vi "Examen2 (2).vi"() -> ()   [LabVIEW 2018]
uses:
  EstadosExamen2.ctl
panel:
  out "Indicador Distancia Recorrida":i32
  out "Indicador Zona Aleatoria":i32
  out "Indicador Nectar Tomado 3":i32(slide) caption="Indicador Salud" scale=0.0..10.0
  out "Indicador Nectar Tomado 2":i32(slide) caption="Indicador Dosis\n       Disponibles" scale=0.0..20.0
  out "Mosca Zona 3":bool
  out "Mosca Zona 2":bool
  out "Mosca Zona 1":bool
  in  "Control Salta":bool
  in  "Control Zona":i32(slide) scale=1.0..3.0
  out "Indicador Zona":i32
  out "Indicador Nectar Tomado":i32(slide) caption="Indicador Nectar\n       Tomado" scale=0.0..5.0
  in  "Control Nectar":bool
  in  "stop":bool
  out "Indicador Estado":T1
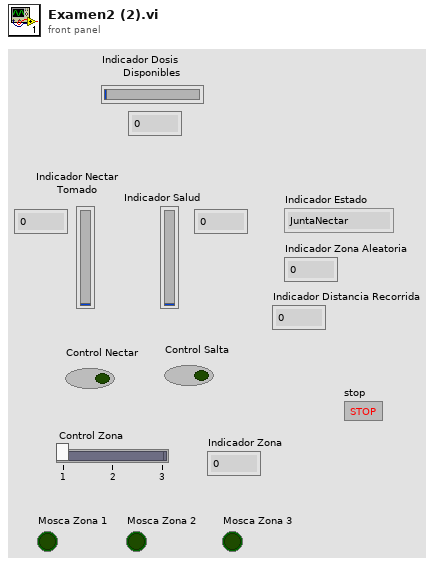
[diagram p1: front panel]
types:
  T1 = typedef "EstadosExamen2.ctl" = enum16{"JuntaNectar", "Volando", "Zona 1", "Zona 2", "Zona 3"}
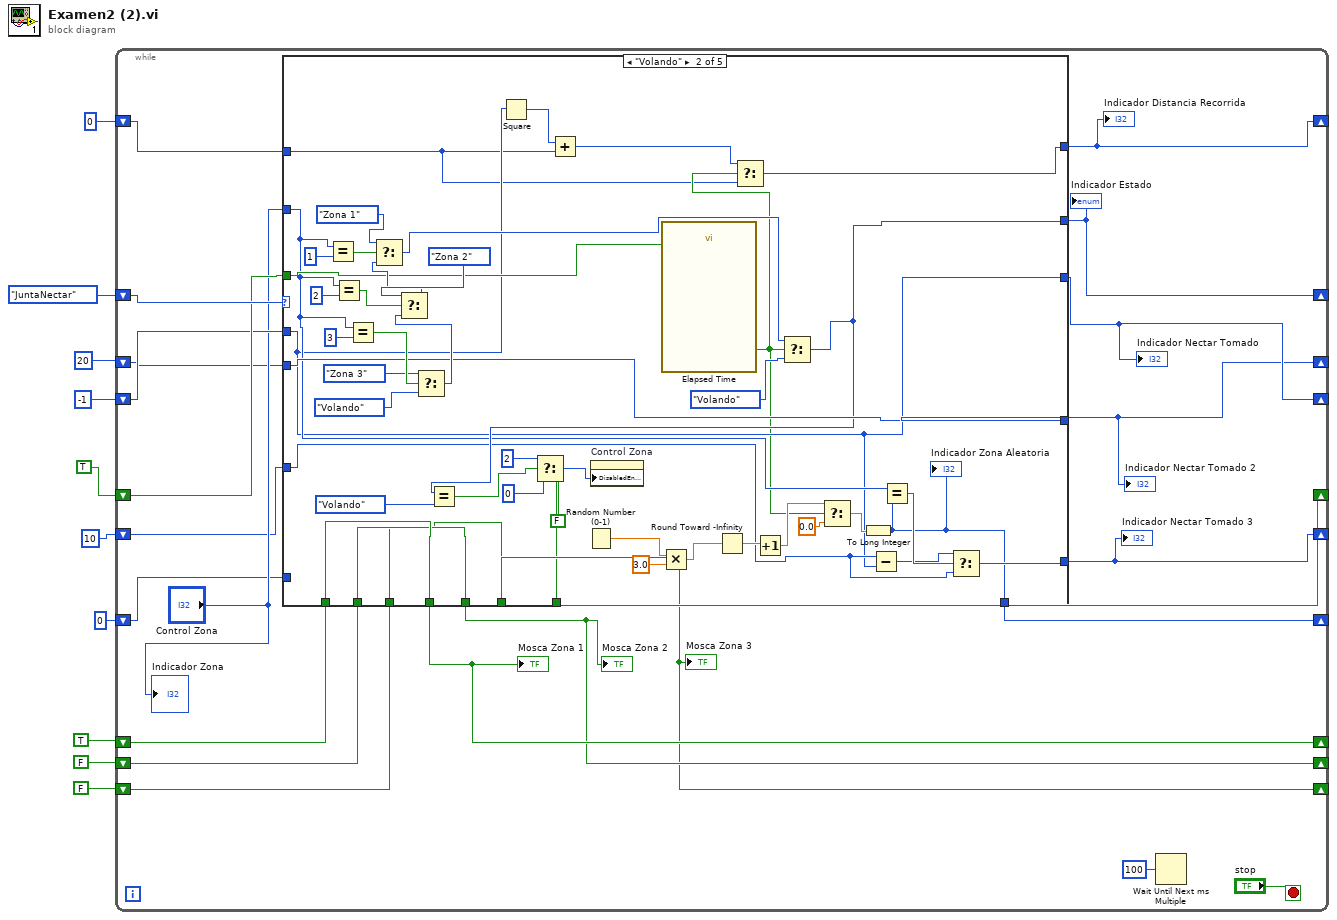
[diagram p0: block diagram]
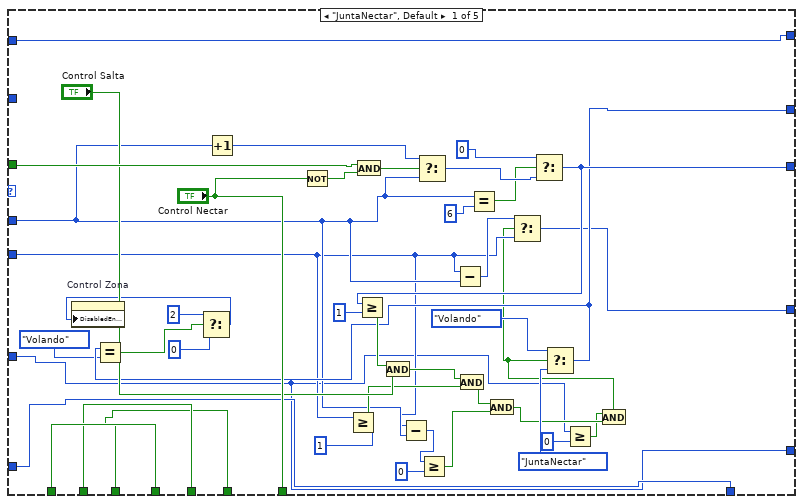
[diagram p2: hidden frame]
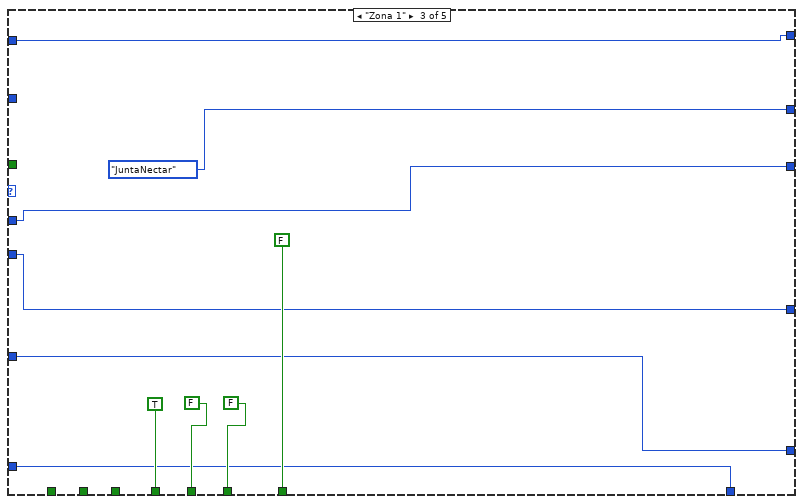
[diagram p3: hidden frame]
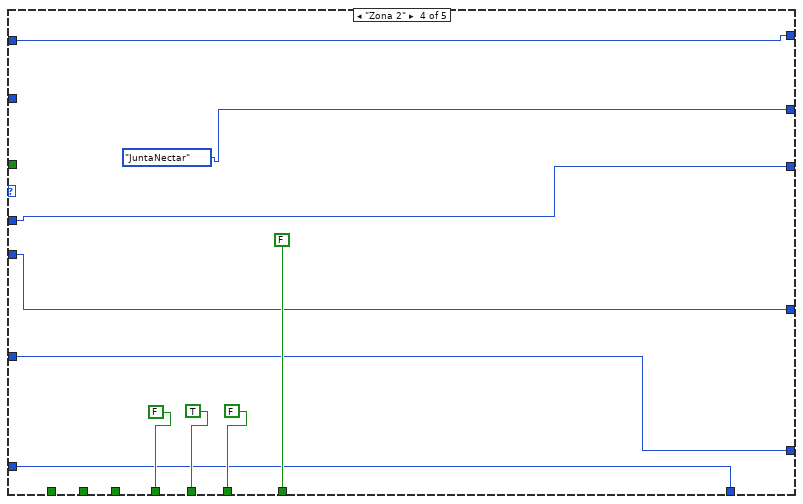
[diagram p4: hidden frame]
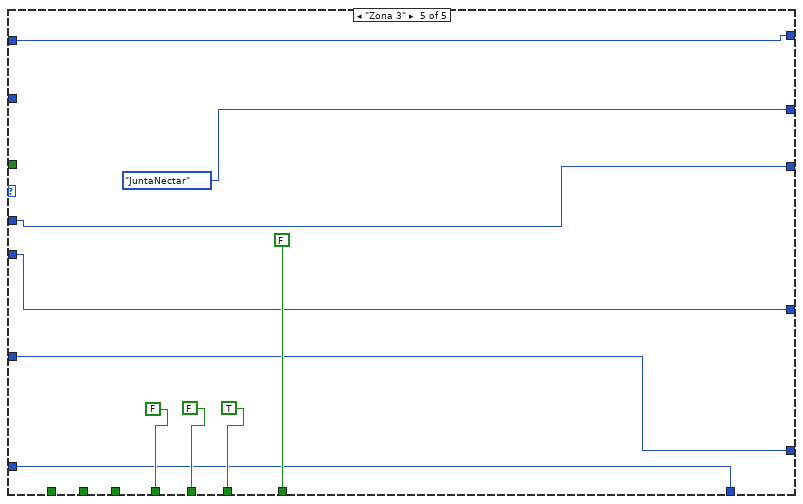
[diagram p5: hidden frame]
diagram:
  n1 = while {
    shift-right: [w32] -> _
    shift-left: EstadosExamen2."JuntaNectar" -> [w33]
    shift-right: [w27] -> _
    shift-left: -1 -> [w26]
    shift-right: [w29] -> _
    shift-left: TRUE -> [w28]
    shift-right: [w21] -> _
    shift-left: TRUE -> [w24]
    shift-right: [w20] -> _
    shift-left: FALSE -> [w23]
    shift-right: [w19] -> _
    shift-left: FALSE -> [w22]
    shift-right: [w18] -> _
    shift-left: 20 -> [w17]
    shift-right: [w15] -> _
    shift-left: 10 -> [w16]
    shift-right: [w14] -> _
    shift-left: 0 -> [w13]
    shift-right: [w11] -> _
    shift-left: 0 -> [w12]
    stop <- "stop" stop-if-true
    n2 = case shown="\"Volando\"" w33 {
      tunnel: [w57 w90 EstadosExamen2."JuntaNectar" EstadosExamen2."JuntaNectar" EstadosExamen2."JuntaNectar"] -> w32
      tunnel: w26 -> [w45 w81 w128 w138 w148]
      tunnel: w28 -> [w68 w98 _ _ _]
      tunnel: [w65 w81 w128 w138 w148] -> w27
      tunnel: ["Control Nectar" FALSE ("Control Nectar 3") FALSE ("Control Nectar 3") FALSE ("Control Nectar 3") FALSE ("Control Nectar 3")] -> w29
      tunnel: "Control Zona" -> [_ w82 _ _ _]
      tunnel: w24 -> [w54 w101 _ _ _]
      tunnel: w23 -> [w53 w100 _ _ _]
      tunnel: w22 -> [w52 w99 _ _ _]
      tunnel: [w54 w101 TRUE FALSE FALSE] -> w21
      tunnel: [w53 w100 FALSE TRUE FALSE] -> w20
      tunnel: [w52 w99 FALSE FALSE TRUE] -> w19
      tunnel: [w41 w97 w124 w134 w144] -> w18
      tunnel: w17 -> [w44 w97 w124 w134 w144]
      tunnel: w16 -> [w35 w84 w123 w133 w143]
      tunnel: [w35 w85 w123 w133 w143] -> w15
      tunnel: [w40 w83 w122 w132 w142] -> w14
      tunnel: w13 -> [w40 _ w122 w132 w142]
      tunnel: w12 -> [w34 w76 w121 w131 w141]
      tunnel: [w34 w77 w121 w131 w141] -> w11
      frame "JuntaNectar", Default {
        n3 = Increment(x=w45) -> (x+1=w73:i32)
        n4 = Not(x="Control Nectar") -> (.not. x?=w71:bool)
        n5 = Greater Or Equal?(x=w44, y=1) -> (x >= y?=w49:bool)
        n6 = And(x=w68, y=w71) -> (x .and. y?=w72:bool)
        n7 = Subtract(x=w44, y=w45) -> (x-y=w43:i32)
        n8 = Select(t=w73, s=w72, f=w45) -> (s? t:f=w75:i32)
        n9 = Greater Or Equal?(x=w43, y=0) -> (x >= y?=w42:bool)
        n10 = Subtract(x=w44, y=w45) -> (x-y=w51:i32)
        n11 = Equal?(x=w45, y=6) -> (x = y?=w74:bool)
        n12 = Select(t=0, s=w74, f=w75) -> (s? t:f=w65:i32)
        n13 = Greater Or Equal?(x=w65, y=1) -> (x >= y?=w63:bool)
        n14 = And(x=w63, y="Control Salta") -> (x .and. y?=w50:bool)
        n15 = And(x=w50, y=w49) -> (x .and. y?=w47:bool)
        n16 = And(x=w47, y=w42) -> (x .and. y?=w39:bool)
        n17 = Greater Or Equal?(x=w35, y=0) -> (x >= y?=w37:bool)
        n18 = And(x=w37, y=w39) -> (x .and. y?=w38:bool)
        n19 = Select(t=w51, s=w38, f=w44) -> (s? t:f=w41:i32)
        n20 = Select(t=EstadosExamen2."Volando", s=w38, f=EstadosExamen2."JuntaNectar") -> (s? t:f=w57:T1)
        n21 = Equal?(x=w57, y=EstadosExamen2."Volando") -> (x = y?=w55:bool)
        n22 = Select(t=2, s=w55, f=0) -> (s? t:f=w58:i32)
        n23 = property on="Control Zona" class="Slide (strict)"("DisabledEnum"=w58) -> ()  [unwired: 2 in, 2 out]
      }
      frame "Volando" {
        n24 = Equal?(x=w82, y=1) -> (x = y?=w115:bool)
        n25 = Equal?(x=w82, y=2) -> (x = y?=w112:bool)
        n26 = Equal?(x=w82, y=3) -> (x = y?=w111:bool)
        n27 = Select(t=EstadosExamen2."Zona 3", s=w111, f=EstadosExamen2."Volando") -> (s? t:f=w107:T1)
        n28 = Select(t=EstadosExamen2."Zona 2", s=w112, f=w107) -> (s? t:f=w108:T1)
        n29 = Select(t=EstadosExamen2."Zona 1", s=w115, f=w108) -> (s? t:f=w89:T1)
        n30 = Square(x=w81) -> (x^2=w80:i32)
        n31 = Add(x=w80, y=w76) -> (x+y=w78:i32)
        n32 = Random Number (0-1)() -> (number: 0 to 1=w93:dbl)
        n33 = Multiply(x=w93, y=3.0) -> (x*y=w94:dbl)
        n34 = call "Elapsed Time"("Reset"=w98) -> ("Time has Elapsed"=w79:bool)  [unwired: 11 in, 7 out]
        n35 = Round Toward -Infinity(1:w94) -> (0:w95:dbl)
        n36 = Select(t=w78, s=w79, f=w76) -> (s? t:f=w77:i32)
        n37 = Increment(x=w95) -> (x+1=w91:dbl)
        n38 = Select(t=w89, s=w79, f=EstadosExamen2."Volando") -> (s? t:f=w90:T1)
        n39 = Equal?(x=w90, y=EstadosExamen2."Volando") -> (x = y?=w104:bool)
        n40 = Select(t=2, s=w104, f=0) -> (s? t:f=w102:i32)
        n41 = property on="Control Zona" class="Slide (strict)"("DisabledEnum"=w102) -> ()  [unwired: 2 in, 2 out]
        n42 = Select(t=w91, s=w79, f=0.0) -> (s? t:f=w88:dbl)
        n43 = To Long Integer(number=w88) -> (32bit integer=w83:i32)
        "Indicador Zona Aleatoria" <- w83
        n44 = Subtract(x=w84, y=w81) -> (x-y=w86:i32)
        n45 = Equal?(x=w82, y=w83) -> (x = y?=w87:bool)
        n46 = Select(t=w86, s=w87, f=w84) -> (s? t:f=w85:i32)
      }
      frame "Zona 1" {
      }
      frame "Zona 2" {
      }
      frame "Zona 3" {
      }
    }
    "Indicador Estado" <- w32
    "Indicador Nectar Tomado" <- w27
    "Mosca Zona 1" <- w21
    "Mosca Zona 2" <- w20
    "Mosca Zona 3" <- w19
    "Indicador Nectar Tomado 2" <- w18
    "Indicador Nectar Tomado 3" <- w15
    "Indicador Distancia Recorrida" <- w11
    n47 = Wait Until Next ms Multiple(millisecond multiple=u32 100) -> ()  [unwired: 1 out]
    "Indicador Zona" <- "Control Zona"
  }
